vi "Test Launcher.vi"() -> ()   [LabVIEW 2022 SP3]
uses:
  Camera Driver/Camera Driver.lvclass
  Camera Controller/Camera Controller.lvclass
  Driver Factories/abstract camera factory/abstract camera driver factory.lvclass
  Camera View/Camera View.lvclass
  36de5d21-3849-4d30-b0a8-b21aec8c176c.vi
  <vilib>/Utility/LVClass/Get LV Class Default Value.vi
  Camera View/Accessors/Write Camera Controller.lvclass.vi
  XY Stage/Framework/Read Configs/Read Configs Sections.lvlib
panel:
  in  "stop":bool
  out "Camera Controller out":refnum<class "Camera Controller.lvclass">
  out "Camera Driver.lvclass":refnum<class "Camera Driver.lvclass">
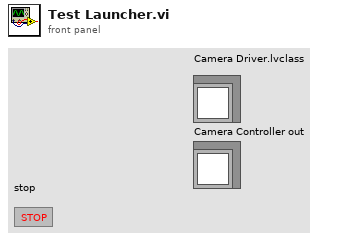
[diagram p1: front panel]
types:
  T1 = typedef "Read Configs Sections.lvlib/Section Data.ctl" = cluster{"Path":path, "Section":string}
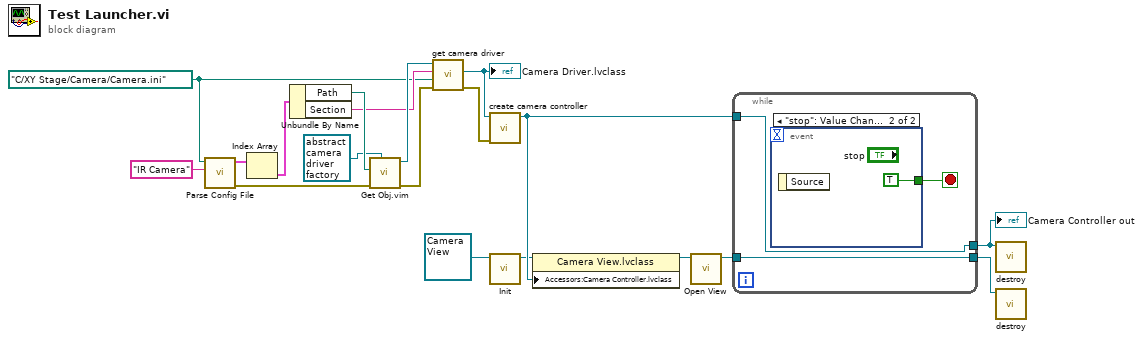
[diagram p0: block diagram]
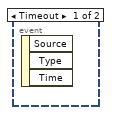
[diagram p2: hidden frame]
diagram:
  w12 = path "C:/XY Stage/Camera/Camera.ini" ("Config Path")
  n1 = call "Parse Config File.vi"("Section"="IR Camera", "Config Path"=w12) -> ("error out"=w11:errorcluster, "Array"=w19:T1[])  [unwired: 8 in]
  n2 = Index Array(array=w19) -> (element=w18:T1)  [unwired: 1 in]
  n3 = Unbundle By Name(w18) -> ("Path"=w16:path, "Section"=w13:string)
  n4 = call "Get Obj.vim"("LabVIEW Object 2"=refnum<class "abstract camera driver factory.lvclass"> refnum ("abstract camera driver factory.lvclass"), "error in (no error)"=w11, "Path"=w16) -> ("error out"=w10:errorcluster, "LabVIEW Object"=w14:refnum<class "abstract camera driver factory.lvclass">)  [unwired: 7 in]
  n5 = call-dynamic "get camera driver.vi"("error in (no error)"=w10, "Path"=w12, "Section"=w13, "abstract camera driver factory in"=w14) -> ("error out"=w8:errorcluster, "Camera Driver.lvclass"=w9:refnum<class "Camera Driver.lvclass">)  [unwired: 6 in]
  "Camera Driver.lvclass" <- w9
  n6 = call "create camera controller.vi"("error in (no error)"=w8, "Camera Driver.lvclass"=w9) -> ("Camera Controller out"=w6:refnum<class "Camera Controller.lvclass">)  [unwired: 8 in, 1 out]
  n7 = call-dynamic "Init.vi"("Camera View in"=refnum<class "Camera View.lvclass"> refnum ("Camera View.lvclass")) -> ("Camera View out"=w4:refnum<class "Camera View.lvclass">)  [unwired: 9 in, 1 out]
  n8 = property class="Camera View.lvclass"(reference=w4, "Accessors:Camera Controller.lvclass"=w6) -> (reference out=w2:refnum<class "Camera View.lvclass">)  [unwired: 1 in, 1 out]
  n9 = call-dynamic "Open View.vi"("base view in"=w2) -> ("base view out"=w1:refnum<class "Camera View.lvclass">)  [unwired: 9 in, 1 out]
  n10 = while {
    tunnel: w6 -> [w21]
    tunnel: [w21] -> w7
    tunnel: w1 -> [w20]
    tunnel: [w20] -> w3
    stop <- w22 stop-if-true
    n11 = event shown="[1] \"stop\": Value Change" {
      selector: _ -> [_ _]
      dyn-events: _ -> [_ _]
      timeout: _ -> [_ _]
      tunnel: [_ TRUE] -> w22
      event Timeout {
        n12 = event-data() -> ()  [unwired: 1 in, 3 out]
      }
      event "stop": Value Change {
        n13 = event-data() -> ()  [unwired: 1 in, 1 out]
      }
    }
  }
  "Camera Controller out" <- w7
  n14 = call-dynamic "destroy.vi"("Camera Controller in"=w7) -> ()  [unwired: 9 in, 2 out]
  n15 = call-dynamic "destroy.vi"("Camera View in"=w3) -> ()  [unwired: 9 in, 2 out]
